vi "MACH_LightDriveCAN.vi"(8 "error in (no error)":errorcluster, 10 "Levels":u8[](array[numeric])) -> (0 "error out":errorcluster, 1 "Bank Trips":bool[](array[boolean]), 2 "Mode":enum8{"NONE", "PWM", "CAN", "SERIAL"}(ring), 3 "Enabled":bool, 4 "Voltage":dbl, 5 "PWM Vals":u8[](array[numeric]), 6 "Currents":dbl[](array[numeric]), 7 "FW Ver":u8)   [LabVIEW 2016]
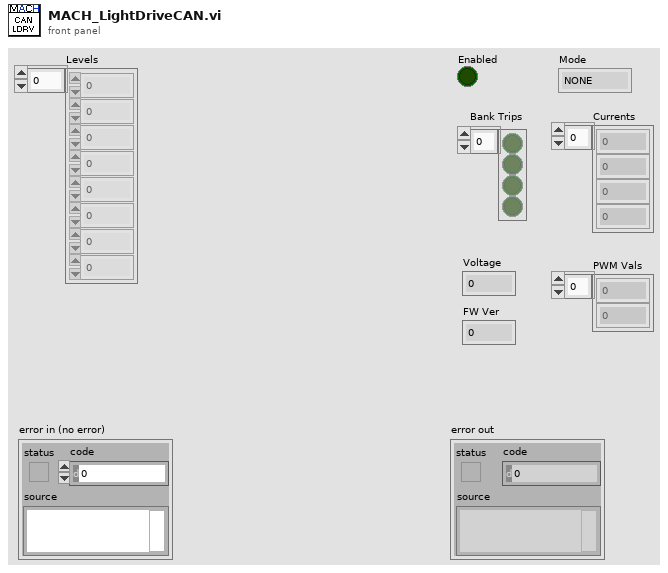
[diagram p1: front panel]
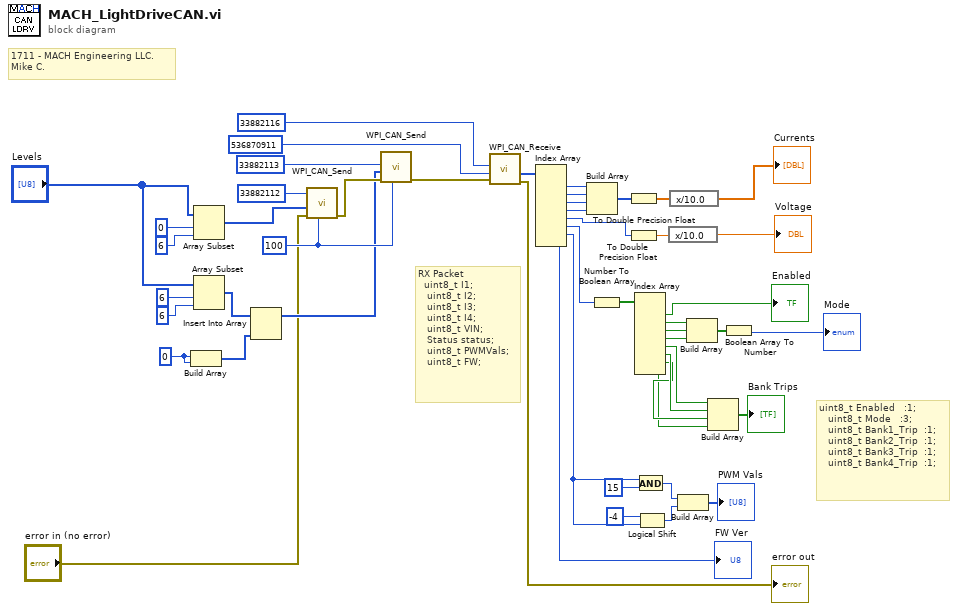
[diagram p0: block diagram]
diagram:
  w40 = u8 0 ("index")
  w49 = 100 ("Period (ms)")
  # "1711 - MACH Engineering LLC.\nMike C."
  # "RX Packet\t\n\t\tuint8_t I1;\n\t\t\tuint8_t I2;\n\t\t\tuint8_t I3;\n\t\t\tuint8_t I4;\n\t\t\tuint8_t VIN;\n\t\t\tStatus status;\n\t\t\tuint8_t PWMVals;\n\t\t\tuint8_t FW;"
  # "uint8_t Enabled\t\t\t:1;\n\t\t\tuint8_t Mode\t\t\t:3;\n\t\t\tuint8_t Bank1_Trip\t\t:1;\n\t\t\tuint8_t Bank2_Trip\t\t:1;\n\t\t\tuint8_t Bank3_Trip\t\t:1;\n\t\t\tuint8_t Bank4_Trip\t\t:1;"
  n1 = Build Array(w40, w40) -> (w41:u8[])
  n2 = Array Subset(array="Levels", index=0, length=6) -> (w38:u8[])
  n3 = Array Subset(array="Levels", index=6, length=6) -> (w42:u8[])
  n4 = Insert Into Array(array=w42, new element=w41) -> (w39:u8[])  [unwired: 1 in]
  n5 = call <vilib>:"WPI_CAN_Send.vi"("Period (ms)"=w49, "error in (no error)"="error in (no error)", "Data"=w38, "Message ID"=u32 33882112) -> ("error out"=w50:errorcluster)  [unwired: 7 in]
  n6 = call <vilib>:"WPI_CAN_Send.vi"("Period (ms)"=w49, "error in (no error)"=w50, "Data"=w39, "Message ID"=u32 33882113) -> ("error out"=w37:errorcluster)  [unwired: 7 in]
  n7 = call <vilib>:"WPI_CAN_Receive.vi"("error in (no error)"=w37, "Message ID Mask"=u32 536870911, "Message ID"=u32 33882116) -> ("error out"=→"error out":errorcluster, "Data"=w34:u8[])  [unwired: 6 in, 1 out]
  n8 = Index Array(array=w34) -> (element #1=w20:u8, element #2=w19:u8, element #3=w18:u8, element #4=w17:u8, element #5=w13:u8, element #6=w21:u8, element #7=w9:u8, element #8=→"FW Ver":u8)  [unwired: 8 in]
  n9 = Build Array(w20, w19, w18, w17) -> (w16:u8[])
  n10 = Number To Boolean Array(number=w21) -> (Boolean array=w33:bool[])
  n11 = To Double Precision Float(number=w16) -> (double precision float=w14:dbl[])
  n12 = To Double Precision Float(number=w13) -> (double precision float=w12:dbl)
  n13 = Index Array(array=w33) -> (element #1=→"Enabled":bool, element #2=w31:bool, element #3=w30:bool, element #4=w29:bool, element #5=w26:bool, element #6=w25:bool, element #7=w24:bool, element #8=w23:bool)  [unwired: 8 in]
  n14 = And(x=w9, y=u8 15) -> (x .and. y?=w7:u8)
  n15 = Logical Shift(y=i16 -4, x=w9) -> (x << y=w6:u8)
  n16 = expression code="x/10.0"(w12) -> (→"Voltage":dbl)
  n17 = expression code="x/10.0"(w14) -> (→"Currents":dbl[])
  n18 = Build Array(w7, w6) -> (→"PWM Vals":u8[])
  n19 = Build Array(w31, w30, w29) -> (w28:bool[])
  n20 = Build Array(w26, w25, w24, w23) -> (→"Bank Trips":bool[])
  n21 = Boolean Array To Number(Boolean array=w28) -> (number=→"Mode":u32)
